vi "Excel Registro.vi"() -> ()   [LabVIEW 2021]
uses:
  <vilib>/Utility/NIReport.llb/Report Type.ctl
  <vilib>/addons/_office/excel.llb/Excel Easy Table (str).vi
  <vilib>/Utility/NIReport.llb/NI_report.lvclass
  <vilib>/addons/_office/NI_ReportGenerationToolkit.lvlib
  <vilib>/Utility/NIReport.llb/NI_ReportGenerationCore.lvlib
  <vilib>/Utility/NIReport.llb/Excel/NI_Excel.lvclass
panel:
  in  "stop":bool
  in  "template (empty)":path
  in  "Iluminidad":dbl(knob) scale=0.0..10.0
  in  "Temperatura":dbl(slide) scale=0.0..100.0
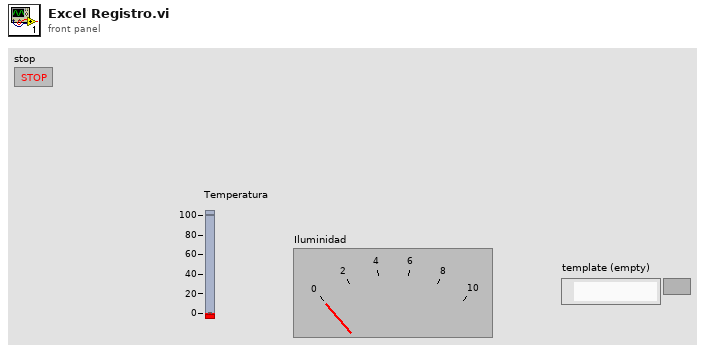
[diagram p1: front panel]
types:
  T1 = typedef "NI_ReportGenerationCore.lvlib/Report Type.ctl" = enum16{"HTML", "Word", "Excel"}
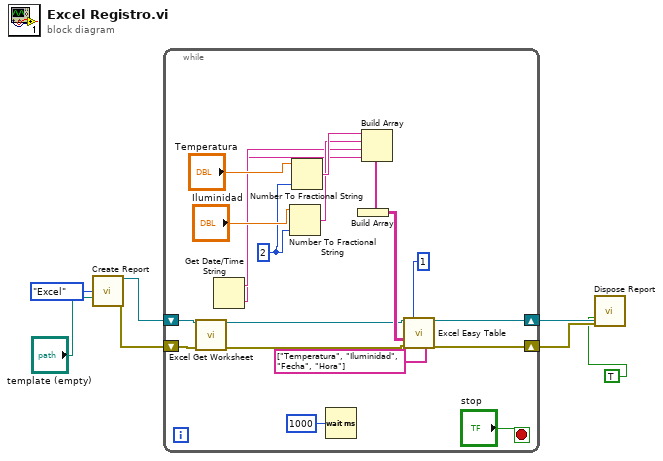
[diagram p0: block diagram]
diagram:
  n1 = call <vilib>:"Create Report.vi"("report type"=Report_Type."Excel", "template (empty)"="template (empty)") -> ("report out"=w4:refnum<class "NI_report.lvclass">, "error out"=w5:errorcluster)  [unwired: 12 in]
  n2 = while {
    shift-right: [w12] -> w2
    shift-left: w5 -> [w17]
    shift-right: [w13] -> w3
    shift-left: w4 -> [w15]
    stop <- "stop" stop-if-true
    w24 = i16 2 ("precision (6)")
    n3 = call <vilib>:"Excel Get Worksheet.vi"("report in"=w15, "error in (no error)"=w17) -> ("report out"=w14:refnum<class "NI_report.lvclass">, "error out"=w16:errorcluster)  [unwired: 12 in]
    n4 = Get Date/Time String() -> (date string=w21:string, time string=w20:string)  [unwired: 3 in]
    n5 = Number To Fractional String(number="Iluminidad", precision (6)=w24) -> (F-format string=w22:string)  [unwired: 2 in]
    n6 = Number To Fractional String(number="Temperatura", precision (6)=w24) -> (F-format string=w23:string)  [unwired: 2 in]
    n7 = Wait (ms)(milliseconds to wait=u32 1000) -> ()  [unwired: 1 out]
    n8 = Build Array(w23, w22, w21, w20) -> (w19:string[])
    n9 = Build Array(w19) -> (w18:string[][])
    n10 = call-poly <vilib>:"Excel Easy Table.vi"("report in"=w14, "iteration"=1, "text data"=w18, "error in (no error)"=w16, "column headers"=string[] ["Temperatura", "Iluminidad", "Fecha", "Hora"]) -> ("report out"=w13:refnum<class "NI_report.lvclass">, "error out"=w12:errorcluster)  [unwired: 6 in, 3 out]
  }
  n11 = call-dynamic "Dispose Report.vi"("report in"=w3, "save changes? (F)"=TRUE, "error in (no error)"=w2) -> ()  [unwired: 12 in, 1 out]
